vi "Actor Core.vi"(8 "error in":errorcluster, 11 "Measure Object in":refnum<class "Rescale.lvclass">) -> (0 "error out":errorcluster, 3 "Actor out":refnum<class "Actor.lvclass">)   [LabVIEW 2018, in "Rescale.lvclass"]
doc: "(<B>Filename</B>: Actor Framework.lvlib:Actor.lvclass:Actor Core.vi)\n\nReceives messages to the actor, reacts to them, and initiates any error handling that may shut the actor down.\n\nDescendant classes may override this VI to append parallel tasks for the actor to complete while it handles messages. Overrides use the Call Parent Method node."
uses:
  Rescale.lvclass
  <vilib>/ActorFramework/Actor/Actor.lvclass
  Rescale Configuration.ctl
  NHMFL_Core/Libraries/File/Controls/NXG TDMS channel re-scale selector entry.ctl
  Process Object/Process Object.lvclass
panel:
  in  "Configuration":T1
  in  "Read channels":bool
  in  "Input file":path
  in  "Re-process":bool
  out "Name":string
  # "Use   Group                     Channel                               New channel                                Scale"
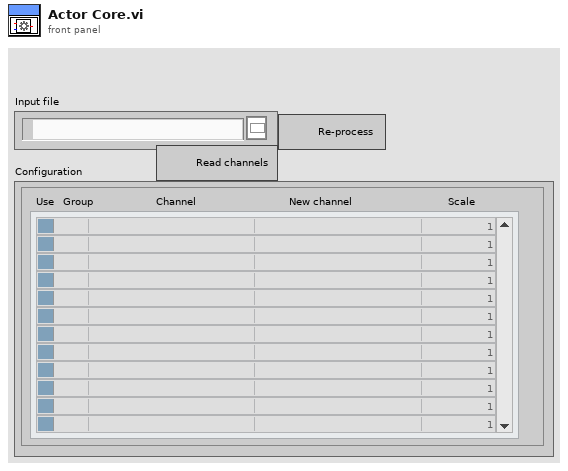
[diagram p1: front panel]
types:
  T1 = typedef "Rescale Configuration.ctl" = cluster{"Channels":T2[]}
  T2 = typedef "NXG TDMS channel re-scale selector entry.ctl" = cluster{"Group":string, "Channel":string, "Active":bool, "New channel":string, "Re-scale factor":dbl}
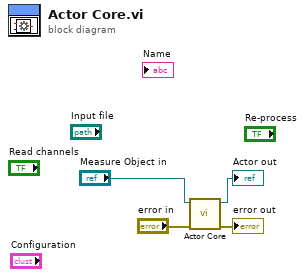
[diagram p0: block diagram]
diagram:
  n1 = call-parent "Actor Core.vi"("error in"="error in", "Measure Object in"="Measure Object in") -> ("error out"=→"error out":errorcluster, "Actor out"=→"Actor out":refnum<class "Actor.lvclass">)  [unwired: 8 in]
